vi "小三轮的 Clock Divisor.vi"(10 "Count Number":u16, 11 "Trigger":bool) -> (3 "Finished":bool)   [LabVIEW 2017]
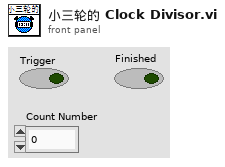
[diagram p1: front panel]
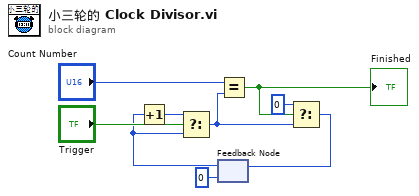
[diagram p0: block diagram]
diagram:
  n1 = feedback #1(u16 0 ("t")) -> (w6:u16)
  n2 = Increment(x=w6) -> (x+1=w1:u16)
  n3 = Select(t=w1, s="Trigger", f=w6) -> (s? t:f=w5:u16)
  n4 = Equal?(x="Count Number", y=w5) -> (x = y?=w4:bool)
  "Finished" <- w4
  n5 = Select(t=u16 0, s=w4, f=w5) -> (s? t:f=w7:u16)
  n6 = feedback-in #1(w7) -> ()
